vi "Rcv Cmd.vi"(8 "error in":errorcluster, 11 "cPAS in":refnum<class "cPAS.lvclass">) -> (0 "error out":errorcluster, 3 "cPAS out":refnum<class "cPAS.lvclass">)   [LabVIEW 2015, in "cPAS.lvclass"]
uses:
  cPAS.lvclass
  Reusable/Instrument/state.ctl
  Reusable/Instrument/Instrument.lvclass
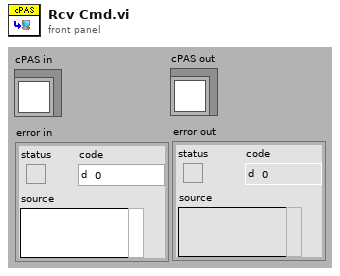
[diagram p1: front panel]
types:
  T1 = typedef "Instrument.lvclass/state.ctl" = enum8{"Configure", "Acquire", "Wait", "Quit", "Handle Error", "NOOP"}
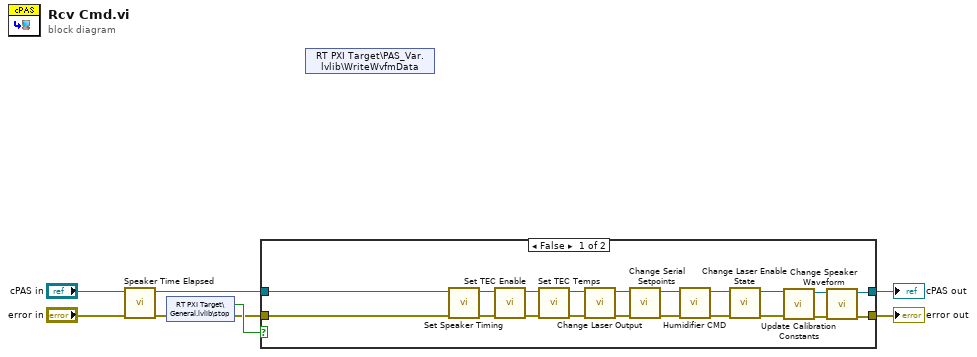
[diagram p0: block diagram]
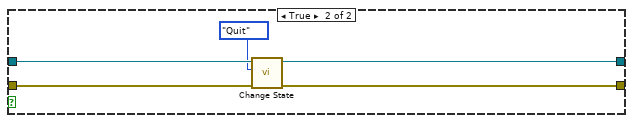
[diagram p2: hidden frame]
diagram:
  n1 = call-dynamic "Speaker Time Elapsed.vi"("error in"="error in", "cPAS in"="cPAS in") -> ("error out"=w1:errorcluster, "cPAS out"=w6:refnum<class "cPAS.lvclass">)  [unwired: 7 in, 1 out]
  n2 = shared-variable "RT PXI Target\\General.lvlib\\stop"(error in=w1) -> (w8:bool, error out=w7:errorcluster)
  n3 = case shown="False" w8 {
    tunnel: w6 -> [w28 w33]
    tunnel: w7 -> [w27 w30]
    tunnel: [w12 w31] -> w4
    tunnel: [w11 w29] -> w3
    frame False {
      n4 = call-dynamic "Set Speaker Timing.vi"("error in"=w27, "cPAS in"=w28) -> ("error out"=w20:errorcluster, "cPAS out"=w18:refnum<class "cPAS.lvclass">)  [unwired: 8 in]
      n5 = call-dynamic "Set TEC Enable.vi"("error in"=w20, "cPAS in"=w18) -> ("error out"=w19:errorcluster, "cPAS out"=w17:refnum<class "cPAS.lvclass">)  [unwired: 8 in]
      n6 = call-dynamic "Set TEC Temps.vi"("error in"=w19, "cPAS in"=w17) -> ("error out"=w24:errorcluster, "cPAS out"=w22:refnum<class "cPAS.lvclass">)  [unwired: 8 in]
      n7 = call-dynamic "Change Laser Output.vi"("error in"=w24, "cPAS in"=w22) -> ("error out"=w23:errorcluster, "cPAS out"=w21:refnum<class "cPAS.lvclass">)  [unwired: 8 in]
      n8 = call "Change Serial Setpoints.vi"("error in"=w23, "cPAS in"=w21) -> ("error out"=w25:errorcluster, "cPAS out"=w26:refnum<class "cPAS.lvclass">)  [unwired: 8 in]
      n9 = call "Humidifier CMD.vi"("error in"=w25, "cPAS in"=w26) -> ("error out"=w9:errorcluster, "cPAS out"=w10:refnum<class "cPAS.lvclass">)  [unwired: 8 in]
      n10 = call "Change Laser Enable State.vi"("error in"=w9, "cPAS in"=w10) -> ("error out"=w15:errorcluster, "cPAS out"=w16:refnum<class "cPAS.lvclass">)  [unwired: 8 in]
      n11 = call "Update Calibration Constants.vi"("error in"=w15, "cPAS in"=w16) -> ("error out"=w13:errorcluster, "cPAS out"=w14:refnum<class "cPAS.lvclass">)  [unwired: 8 in]
      n12 = call "Change Speaker Waveform.vi"("error in"=w13, "cPAS in"=w14) -> ("error out"=w11:errorcluster, "cPAS out"=w12:refnum<class "cPAS.lvclass">)  [unwired: 8 in]
    }
    frame True {
      n13 = call "Change State.vi"("error in"=w30, "instr state"=state."Quit", "Instrument in"=w33) -> ("error out"=w29:errorcluster, "Instrument out"=w31:refnum<class "cPAS.lvclass">)  [unwired: 7 in]
    }
  }
  "error out" <- w3
  "cPAS out" <- w4
  n14 = shared-variable "RT PXI Target\\PAS_Var.lvlib\\WriteWvfmData"() -> ()  [unwired: 1 in, 2 out]
